vi "Motor.vi"(2 "error in":errorcluster, 3 "Motor on?":bool, 4 "Serial Port in":refnum<visa-resource-name>) -> (0 "error out":errorcluster, 1 "Serial Port out":refnum<visa-resource-name>)   [LabVIEW 2011]
doc: "Sends commands for turning the motor on or off to the Arduino."
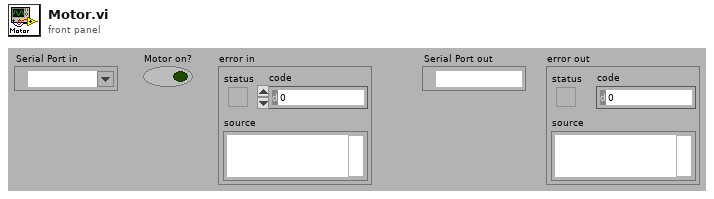
[diagram p1: front panel]
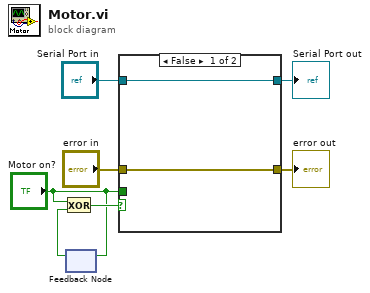
[diagram p0: block diagram]
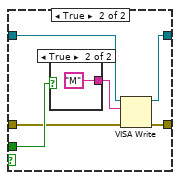
[diagram p2: hidden frame]
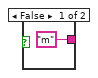
[diagram p3: hidden frame]
diagram:
  n1 = feedback #1() -> (w2:bool)  [unwired: 1 in]
  n2 = Exclusive Or(1:w2, 2:"Motor on?") -> (0:w3:bool)
  n3 = feedback-in #1("Motor on?") -> ()
  n4 = case shown="False" w3 {
    tunnel: "Motor on?" -> [_ w14]
    tunnel: "Serial Port in" -> [w8 w13]
    tunnel: "error in" -> [w9 w12]
    tunnel: [w9 w11] -> w5
    tunnel: [w8 w10] -> w7
    frame False {
    }
    frame True {
      n5 = case shown="True" w14 {
        tunnel: ["m" "M"] -> w15
        frame False {
        }
        frame True {
        }
      }
      n6 = VISA Write(VISA resource name=w13, write buffer=w15, error in (no error)=w12) -> (VISA resource name out=w10:refnum<visa-resource-name>, error out=w11:errorcluster)  [unwired: 1 out]
    }
  }
  "Serial Port out" <- w7
  "error out" <- w5
